vi "Handle Error.vi"(7 "Websocket Client Handler in":refnum<class "Websocket Client Handler.lvclass">, 8 "error in (no error)":errorcluster) -> (0 "error out":errorcluster, 3 "Stop Actor?":bool, 5 "Websocket Client Handler out":refnum<class "Websocket Client Handler.lvclass">)   [LabVIEW 2016, in "Stream Mediator.lvlib" / "Websocket Client Handler.lvclass"]
doc: "--\nCopyright © 2017 Composed SystemsI All rights reserved.\n\nAuthor: Jon McBee <jon.mcbee@composed.io>\n\nThis library is provided \"AS IS\" ,WITHOUT WARRANTIES OR\nCONDITIONS OF ANY KIND, either express or implied.\n\nComposed Systems -- composed.io\n\nStream 0.0.1.1\nJon McBee - Composed Systems\nCopyright (c) 2017, Composed Systems"
uses:
  <userlib>/Composed Systems/Stream/Mediator/Classes/Websocket Client Handler Actor/Websocket Client Handler/Websocket Client Handler.lvclass
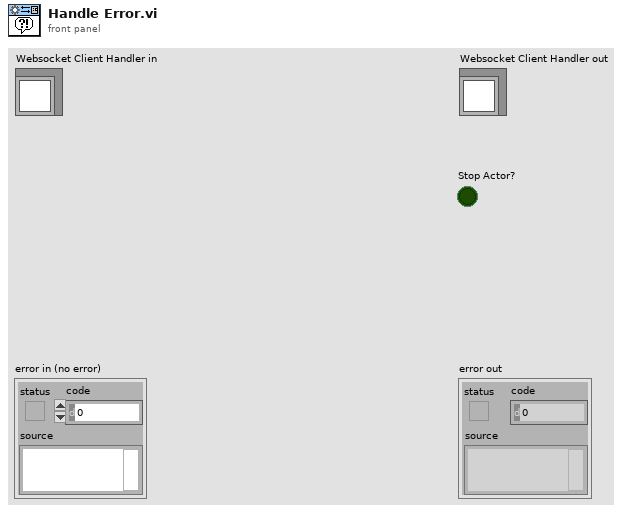
[diagram p1: front panel]
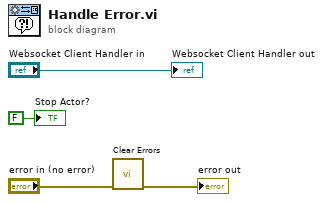
[diagram p0: block diagram]
diagram:
  n1 = call <vilib>:"Clear Errors.vi"("error in (no error)"="error in (no error)") -> ("error out"=→"error out":errorcluster)  [unwired: 5 in, 1 out]
  "Websocket Client Handler out" <- "Websocket Client Handler in"
  "Stop Actor?" <- FALSE ("Stop Actor?")
